vi "Do.vi"(8 "error in (no error)":errorcluster, 10 "Actor in":refnum<class "Actor.lvclass">, 11 "tt20panel_DO_stream_data Msg":refnum<class "tt20panel_DO_stream_data Msg.lvclass">) -> (0 "error out":errorcluster, 2 "Actor out":refnum<class "Actor.lvclass">)   [LabVIEW 2015, in "tt20panel_DO_stream_data Msg.lvclass"]
doc: "This VI delivers the message to the actor by calling the appropriate method(s) on the actor."
uses:
  tt20panel_DO_stream_data Msg.lvclass
  <vilib>/ActorFramework/Actor/Actor.lvclass
  tt20panel_class/tt20panel.lvclass
  tt20panel_DO_stream_data Msg.lvclass/tt20panel_DO_stream_data Msg.ctl
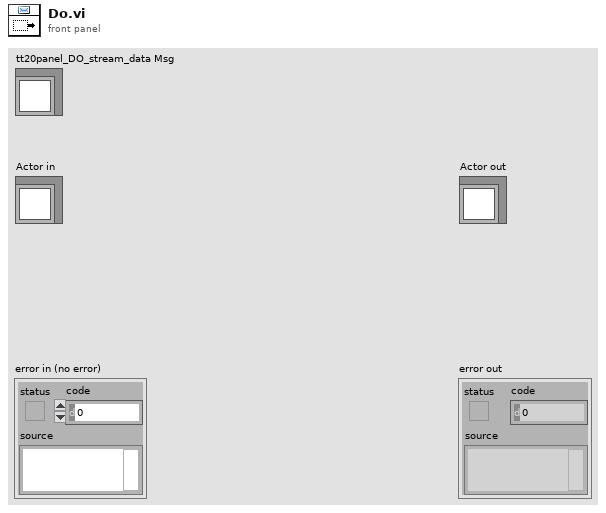
[diagram p1: front panel]
types:
  T1 = typedef "tt20_stream_settings_tdef.ctl" = cluster{"Stream Path":path, "acq_time (s)":u32, "Stream Notes":string}
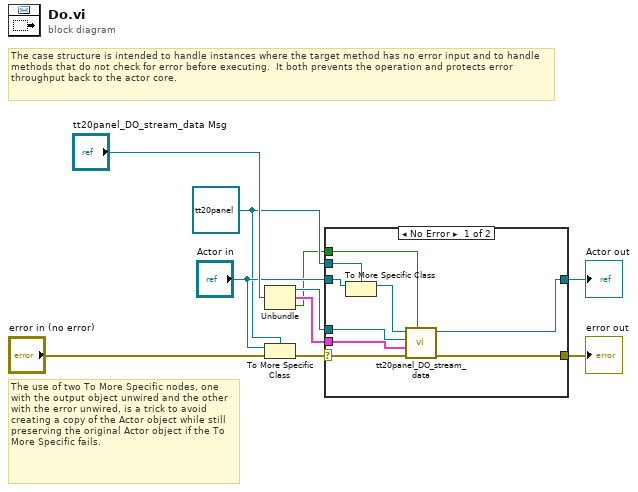
[diagram p0: block diagram]
diagram:
  w4 = refnum<class "tt20panel.lvclass"> refnum ("Actor in")
  # "The use of two To More Specific nodes, one with the output object unwired and the other with the error unwired, is a trick to avoid creating a copy of the Actor object while still preserving the original Actor object if the To More Specific fails."
  # "The case structure is intended to handle instances where the target method has no error input and to handle methods that do not check for error before executing.  It both prevents the operation and protects error throughput back to the actor core."
  n1 = Unbundle("tt20panel_DO_stream_data Msg") -> (w3:refnum<queue>, w2:T1, w1:bool)
  n2 = To More Specific Class(target class=w4, reference="Actor in", error in="error in (no error)") -> (error out=w8:errorcluster)  [unwired: 1 out]
  n3 = case shown="No Error" w8 {
    selector: w8 -> [w17 w21]
    tunnel: [w19 w21] -> w7
    tunnel: [w18 w20] -> w6
    tunnel: "Actor in" -> [w16 w20]
    tunnel: w4 -> [w15 _]
    tunnel: w3 -> [w13 _]
    tunnel: w2 -> [w12 _]
    tunnel: w1 -> [w11 _]
    frame No Error {
      n4 = To More Specific Class(target class=w15, reference=w16) -> (specific class reference=w14:refnum<class "tt20panel.lvclass">)  [unwired: 1 in, 1 out]
      n5 = call "tt20panel_DO_stream_data.vi"("Overwrite?"=w11, "error in (no error)"=w17, "stream_settings"=w12, "stop_counts"=w13, "tt20panel in"=w14) -> ("error out"=w19:errorcluster, "tt20panel out"=w18:refnum<class "tt20panel.lvclass">)  [unwired: 5 in]
    }
    frame Error {
      # "If type check fails, pass the original object out again."
    }
  }
  "error out" <- w7
  "Actor out" <- w6
